vi "WriteLedArray.vi"(8 "error in (no error)":errorcluster, 9 "LED Colors":u32[](array[colorbox]), 10 "Chains":u8[](array[numeric]), 11 "ControlState in":T2 {"ChainMask" format="0x%02x"}) -> (0 "error out":errorcluster, 3 "ControlState out":T2 {"ChainMask" format="0x%02x"}, 5 "Optimization":T1)   [LabVIEW 2023, in "ArduinoSerialBling.lvlib"]
uses:
  ArduinoSerialBling.lvlib
  ControlState.ctl
  ConnectionType.ctl
  UdpConnection.ctl
  ChainState.ctl
  WriteLedArrayStatus.ctl
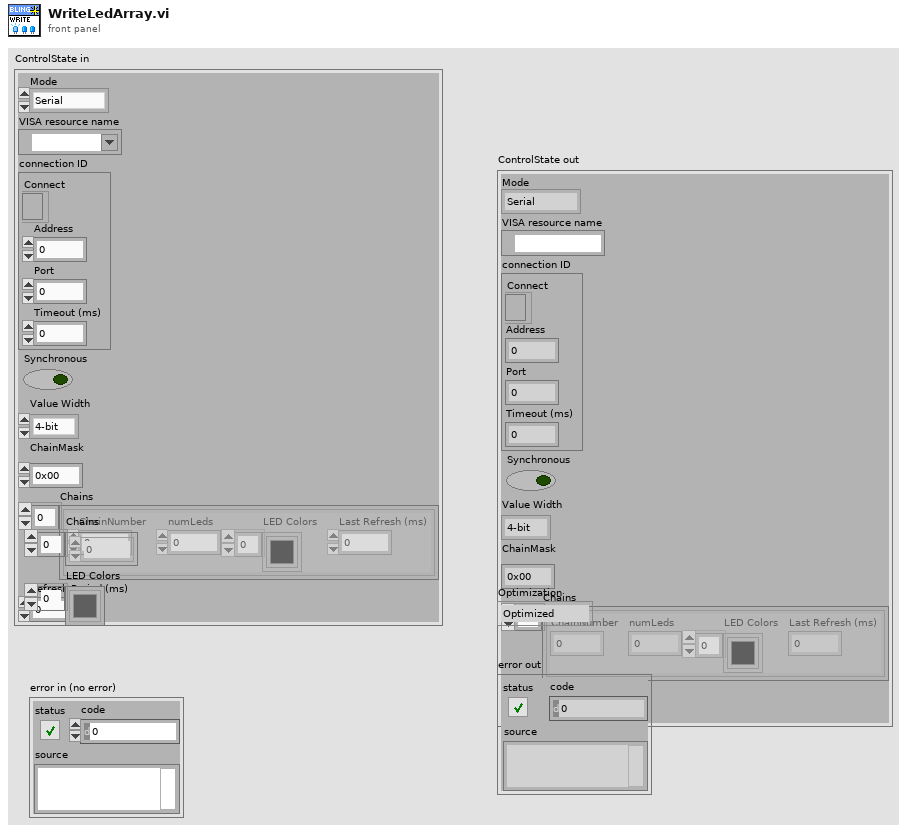
[diagram p1: front panel]
types:
  T1 = typedef "ArduinoSerialBling.lvlib/WriteLedArrayStatus.ctl" = enum16{"Optimized", "Unable to optimize", "No changes", "Error", "Offline"}
  T2 = typedef "ArduinoSerialBling.lvlib/ControlState.ctl" = cluster{"Mode":T3, "VISA resource name":refnum<visa-resource-name>, "connection ID":T4, "Synchronous":bool, "Value Width":enum16{"4-bit", "8-bit"}, "ChainMask":u8, "Chains":T5[], "Refresh Period (ms)":u32}
  T3 = typedef "ConnectionType.ctl" = enum16{"Serial", "Ethernet", "Offline"}
  T4 = typedef "UdpConnection.ctl" = cluster{"Connect":refnum<k16>, "Address":u32, "Port":u16, "Timeout (ms)":i32}
  T5 = typedef "ArduinoSerialBling.lvlib/ChainState.ctl" = cluster{"ChainNumber":u8, "numLeds":u8, "LED Colors":u32[], "Last Refresh (ms)":u32}
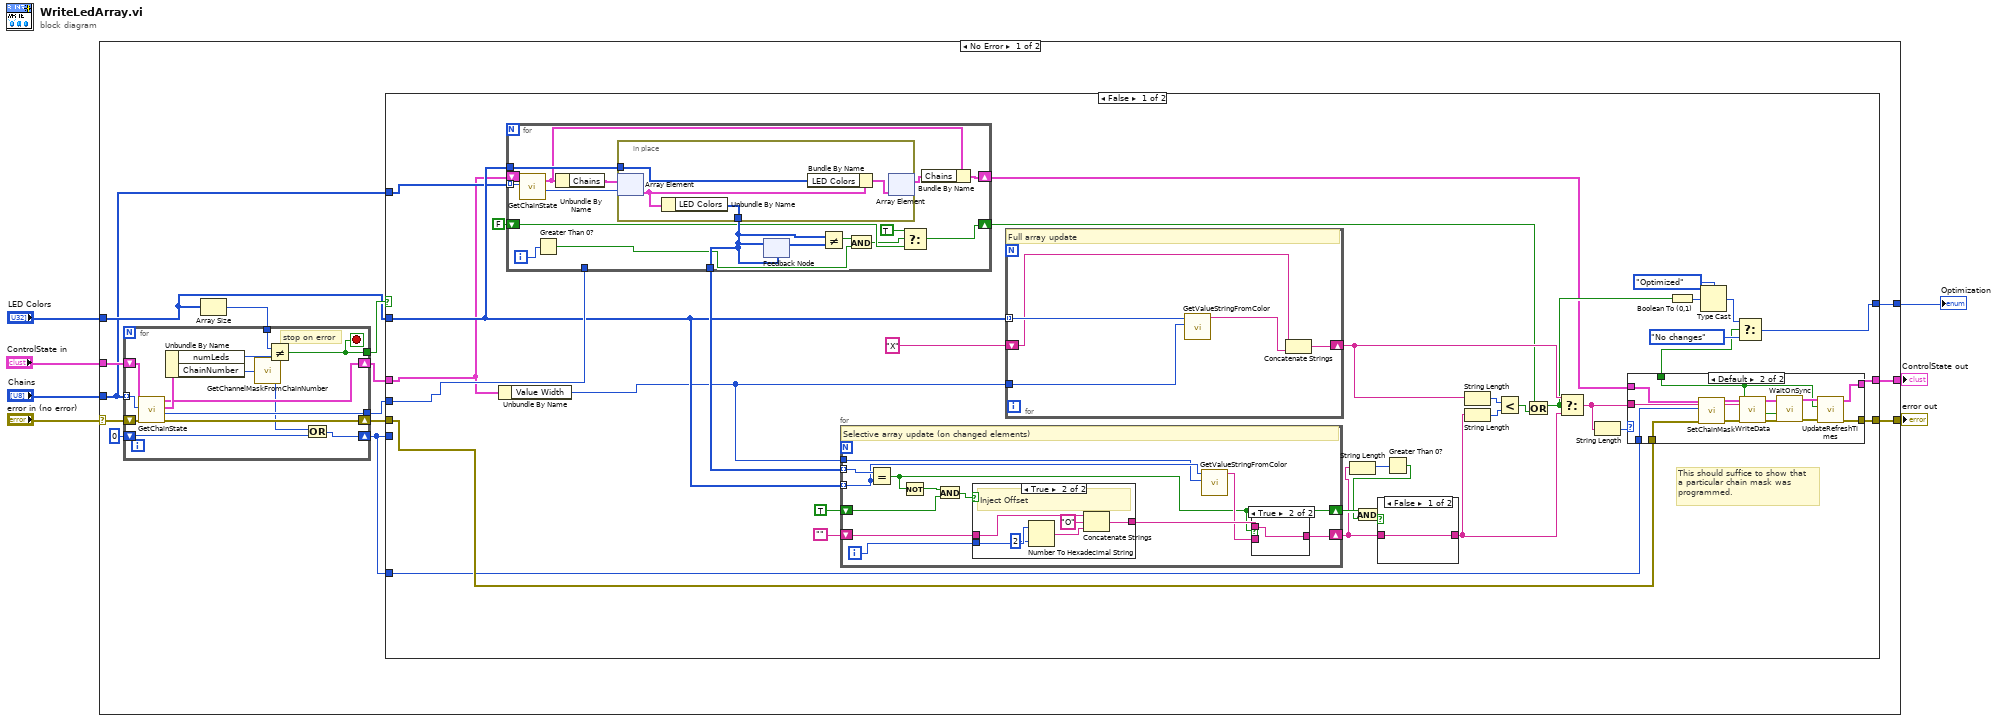
[diagram p0: block diagram]
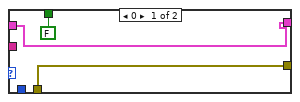
[diagram p2: hidden frame]
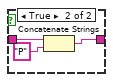
[diagram p3: hidden frame]
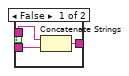
[diagram p4: hidden frame]
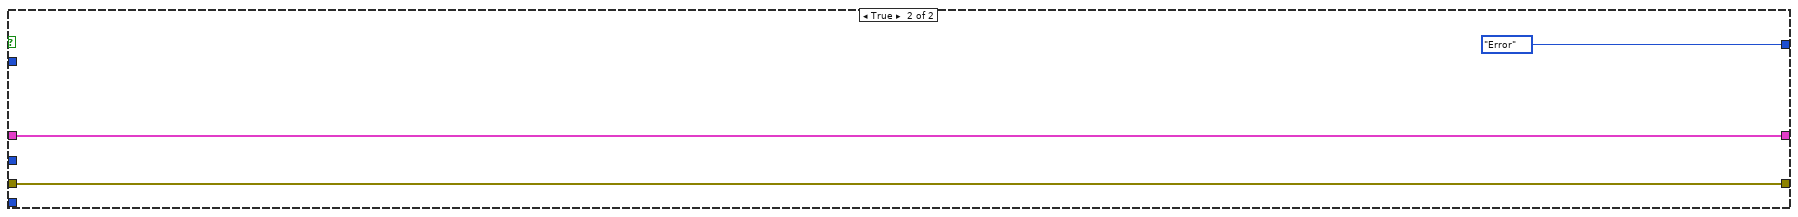
[diagram p6: hidden frame]
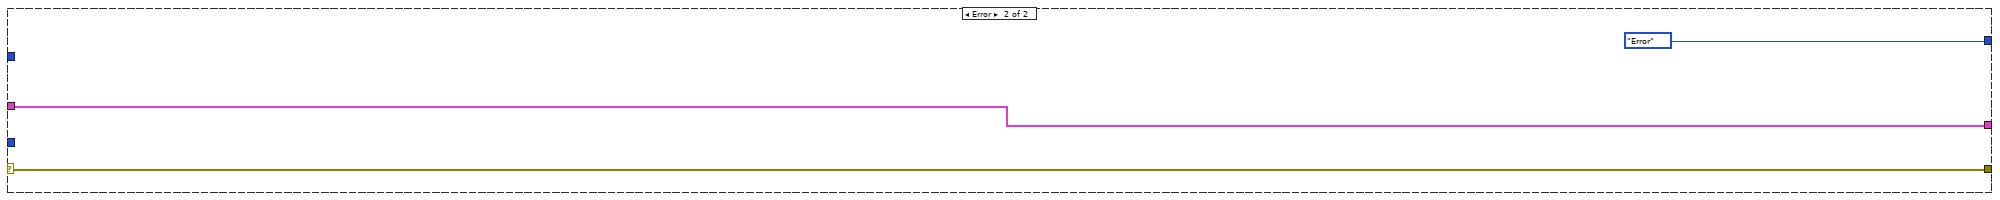
[diagram p7: hidden frame]
diagram:
  n1 = case shown="No Error" "error in (no error)" {
    selector: "error in (no error)" -> [w13 w145]
    tunnel: [w18 w145] -> w7
    tunnel: [w19 w143] -> w6
    tunnel: "LED Colors" -> [w20 _]
    tunnel: [w17 WriteLedArrayStatus."Error" ("Optimization")] -> w4
    tunnel: "ControlState in" -> [w16 w143]
    tunnel: "Chains" -> [w9 _]
    frame No Error {
      n2 = Array Size(array=w20) -> (size(s)=w12:i32)
      n3 = for {
        tunnel: [w26] -> w21
        tunnel: [w34] -> w15
        tunnel: w12 -> [w29]
        shift-right: [w32] -> w14
        shift-left: w16 -> [w35]
        shift-right: [w28] -> w11
        shift-left: w13 -> [w31]
        tunnel: w9 -> [w27] mode=indexing
        shift-right: [w22] -> w8
        shift-left: u8 0 -> [w23]
        stop <- w26 stop-if-true
        # "stop on error"
        n4 = call "GetChainState.vi"("error in (no error)"=w31, "ChainNumber"=w27, "ControlState in"=w35) -> ("error out"=w28:errorcluster, "ChainIndex"=w34:i32, "ChainState"=w33:T5, "ControlState out"=w32:T2)  [unwired: 5 in]
        n5 = Unbundle By Name(w33) -> ("numLeds"=w30:u8, "ChainNumber"=w25:u8)
        n6 = call "GetChannelMaskFromChainNumber.vi"("ChainNumber"=w25) -> ("ChainMask"=w24:u8)
        n7 = Not Equal?(x=w29, y=w30) -> (x != y?=w26:bool)
        n8 = Or(x=w24, y=w23) -> (x .or. y?=w22:u8)
      }
      n9 = case shown="False" w21 {
        tunnel: w11 -> [w39 w141]
        tunnel: w14 -> [w40 w142]
        tunnel: w20 -> [w64 _]
        tunnel: w15 -> [w70 _]
        tunnel: [w42 w142] -> w19
        tunnel: [w41 w141] -> w18
        tunnel: [w51 WriteLedArrayStatus."Error" ("Optimization")] -> w17
        tunnel: w8 -> [_ _]
        tunnel: w9 -> [w49 _]
        tunnel: w8 -> [w36 _]
        frame False {
          # "This should suffice to show that\na particular chain mask was\nprogrammed."
          n10 = Unbundle By Name(w40) -> ("Value Width"=w61:enum16{"4-bit", "8-bit"})
          n11 = for {
            tunnel: w70 -> [_]
            tunnel: [w97] -> w65
            tunnel: w64 -> [w103]
            tunnel: w49 -> [w102] mode=indexing
            shift-right: [w94] -> w45
            shift-left: FALSE -> [w96]
            shift-right: [w92] -> w44
            shift-left: w40 -> [w101]
            i -> [w90]
            n12 = call "GetChainState.vi"("ChainNumber"=w102, "ControlState in"=w101) -> ("ChainIndex"=w100:i32, "ControlState out"=w93:T2)  [unwired: 6 in, 2 out]
            n13 = Greater Than 0?(x=w90) -> (x > 0?=w88:bool)
            n14 = Unbundle By Name(w93) -> ("Chains"=w99:T5[])
            n15 = in-place {
              in-place-border: w103 -> [w106]
              in-place-border: [w104] -> w97
              n16 = in-place-array #1(w99, w100) -> (w105:T5)
              n17 = Unbundle By Name(w105) -> ("LED Colors"=w104:u32[])
              n18 = Bundle By Name(cluster=w105, "LED Colors"=w106) -> (w107:T5)
              n19 = in-place-array #1(w107) -> (w91:T5[])  [unwired: 1 out]
            }
            n20 = feedback-in #2(w97) -> ()
            n21 = feedback #2(w97) -> (w98:u32[])
            n22 = Not Equal?(x=w97, y=w98) -> (x != y?=w89:bool)
            n23 = And(x=w89, y=w88) -> (x .and. y?=w87:bool)
            n24 = Select(t=TRUE, s=w87, f=w96) -> (s? t:f=w94:bool)
            n25 = Bundle By Name(cluster=w93, "Chains"=w91) -> (w92:T2)
          }
          n26 = for {
            tunnel: w65 -> [w123] mode=indexing
            tunnel: w64 -> [w117] mode=indexing
            shift-right: [w112] -> w56
            shift-left: TRUE -> [w122]
            shift-right: [w113] -> w55
            shift-left: "" -> [w118]
            tunnel: w61 -> [w116]
            i -> [w119]
            # "Selective array update (on changed elements)"
            n27 = Equal?(x=w123, y=w117) -> (x = y?=w112:bool)
            n28 = Not(x=w112) -> (.not. x?=w121:bool)
            n29 = And(x=w121, y=w122) -> (x .and. y?=w120:bool)
            n30 = case shown="True" w120 {
              tunnel: w119 -> [_ w132]
              tunnel: w118 -> [w128 w134]
              tunnel: [w128 w129] -> w115
              frame False {
                # "Continue inserting values"
              }
              frame True {
                # "Inject Offset"
                n31 = Number To Hexadecimal String(1:i16 2 ("width (-)"), 2:w132) -> (0:w130:string)
                n32 = Concatenate Strings(w134, "O" ("string"), w130) -> (w129:string)
              }
            }
            n33 = call "GetValueStringFromColor.vi"("Value Width"=w116, "Color"=w117) -> ("Value String"=w114:string)  [unwired: 9 in]
            n34 = case shown="True" w112 {
              tunnel: w115 -> [w126 w127]
              tunnel: w114 -> [w125 _]
              tunnel: [w124 w127] -> w113
              frame False {
                n35 = Concatenate Strings(w126, w125) -> (w124:string)
              }
              frame True {
              }
            }
          }
          n36 = for {
            tunnel: w64 -> [w139] mode=indexing
            shift-right: [w136] -> w67
            shift-left: "X" -> [w138]
            tunnel: w61 -> [w135]
            # "Full array update"
            n37 = call "GetValueStringFromColor.vi"("Value Width"=w135, "Color"=w139) -> ("Value String"=w137:string)  [unwired: 9 in]
            n38 = Concatenate Strings(w138, w137) -> (w136:string)
          }
          n39 = String Length(string=w55) -> (length=w54:i32)
          n40 = Greater Than 0?(x=w54) -> (x > 0?=w53:bool)
          n41 = And(x=w56, y=w53) -> (x .and. y?=w57:bool)
          n42 = case shown="False" w57 {
            tunnel: w55 -> [w108 w111]
            tunnel: [w108 w109] -> w60
            frame False {
            }
            frame True {
              n43 = Concatenate Strings(w111, "P" ("string")) -> (w109:string)
            }
          }
          n44 = String Length(string=w67) -> (length=w68:i32)
          n45 = String Length(string=w60) -> (length=w66:i32)
          n46 = Less?(x=w68, y=w66) -> (x < y?=w46:bool)
          n47 = Or(x=w45, y=w46) -> (x .or. y?=w47:bool)
          n48 = Select(t=w67, s=w47, f=w60) -> (s? t:f=w37:string)
          n49 = String Length(string=w37) -> (length=w38:i32)
          n50 = case shown="Default" w38 {
            tunnel: w39 -> [w71 w75]
            tunnel: w37 -> [_ w84]
            tunnel: w44 -> [w72 w74]
            tunnel: [FALSE ("Data Written?") w81] -> w43
            tunnel: [w72 w80] -> w42
            tunnel: [w71 w79] -> w41
            tunnel: w36 -> [_ w78]
            frame 0 {
            }
            frame Default {
              n51 = call "SetChainMask.vi"("error in (no error)"=w75, "ChainMask"=w78, "ControlState in"=w74) -> ("error out"=w76:errorcluster, "ControlState out"=w77:T2)  [unwired: 7 in]
              n52 = call "WriteData.vi"("error in (no error)"=w76, "Command"=w84, "ControlState in"=w77) -> ("error out"=w86:errorcluster, "Data Written?"=w81:bool, "ControlState out"=w85:T2)  [unwired: 5 in, 1 out]
              n53 = call "WaitOnSync.vi"("error in (no error)"=w86, "Enable"=w81, "ControlState in"=w85) -> ("error out"=w82:errorcluster, "ControlState out"=w83:T2)  [unwired: 7 in]
              n54 = call "UpdateRefreshTimes.vi"("error in (no error)"=w82, "Update Time"=w81, "ControlState in"=w83) -> ("error out"=w79:errorcluster, "ControlState out"=w80:T2)  [unwired: 7 in]
            }
          }
          n55 = Boolean To (0,1)(Boolean=w47) -> (0, 1=w58:i16)
          n56 = Type Cast(type=WriteLedArrayStatus."Optimized" ("Optimization"), x=w58) -> (*(type *) &x=w52:T1)
          n57 = Select(t=w52, s=w43, f=WriteLedArrayStatus."No changes") -> (s? t:f=w51:T1)
        }
        frame True {
        }
      }
    }
    frame Error {
    }
  }
  "ControlState out" <- w6
  "error out" <- w7
  "Optimization" <- w4
